vi "SequenceVI.vi"(5 "MSComm":refnum<k7>, 6 "semaphore":T1 caption="信号量", 7 "GUIRefArray":T3[](array[typedef]), 8 "error in":errorcluster, 9 "Slot":T2, 10 "SlotEnable":enum16{"Enable", "Disable"}(ring)=enum."Disable", 11 "QueueArray":variant[](array[variant])) -> (0 "error out":errorcluster)   [LabVIEW 2013]
uses:
  SystemCode/SysControl/Reference.ctl
  SystemCode/SysControl/TestItemsCTL.ctl
  SystemCode/SysControl/Slot.ctl
  SystemCode/SysControl/States.ctl
  SystemCode/DeStateQueue.vi
  SystemCode/EnStateQueue.vi
  SystemCode/ReleaseStateQueue.vi
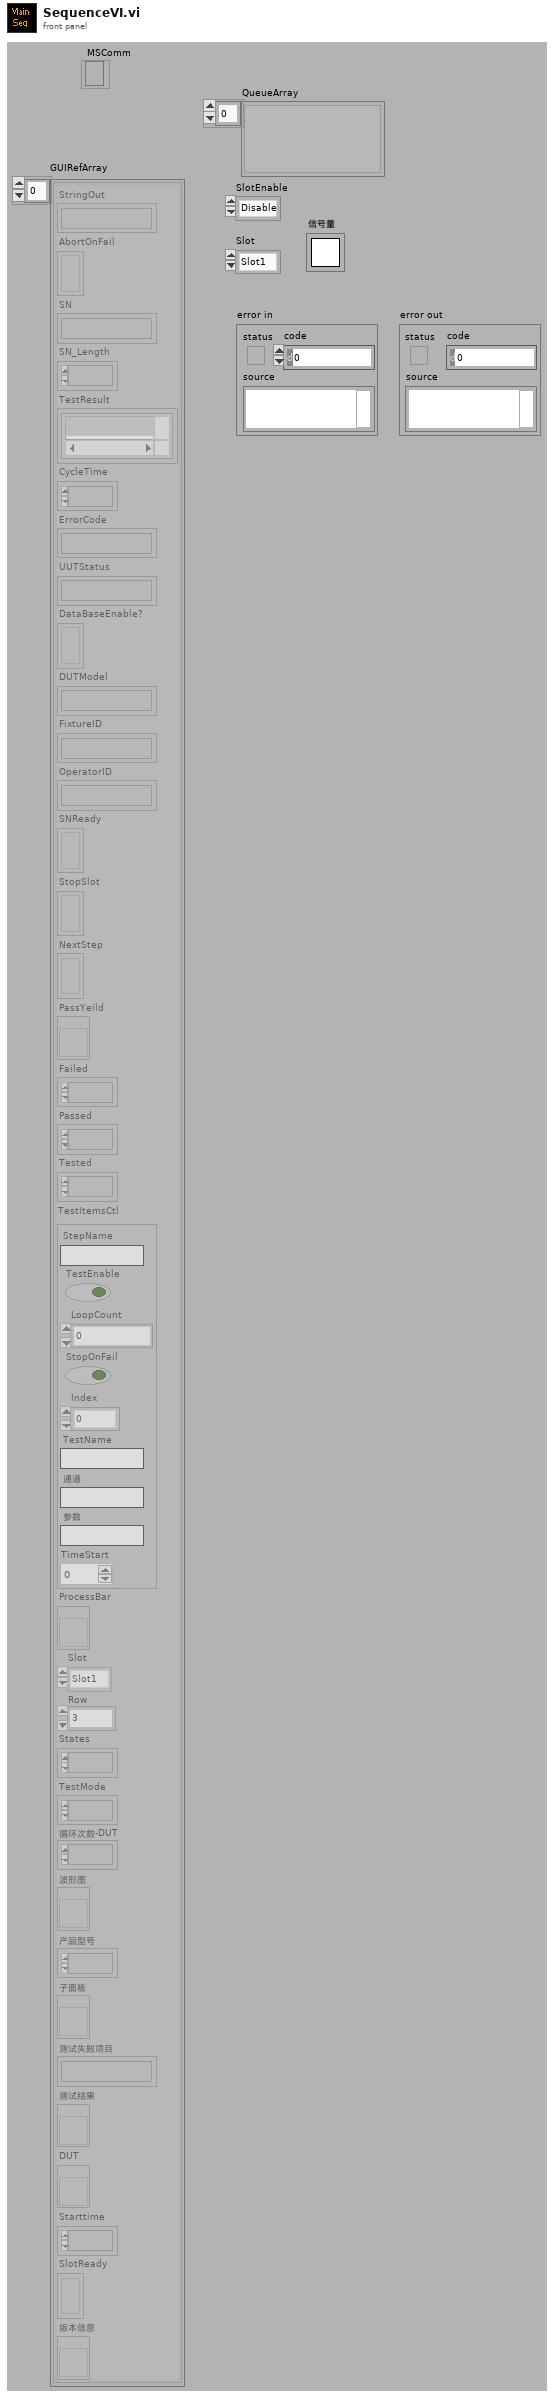
[diagram p1: front panel]
types:
  T1 = typedef "Semaphore RefNum" = refnum<k1>
  T2 = typedef "Slot.ctl" = enum16{"Slot1", "Slot2", "Slot3", "Slot4"}
  T3 = typedef "Reference.ctl" = cluster{"StringOut":refnum<vi>, "AbortOnFail":refnum<vi>, "SN":refnum<vi>, "SN_Length":refnum<vi>, "TestResult":refnum<vi>, "CycleTime":refnum<vi>, "ErrorCode":refnum<vi>, "UUTStatus":refnum<vi>, "DataBaseEnable?":refnum<vi>, "DUTModel":refnum<vi>, "FixtureID":refnum<vi>, "OperatorID":refnum<vi>, "SNReady":refnum<vi>, "StopSlot":refnum<vi>, "NextStep":refnum<vi>, "PassYeild":refnum<vi>, "Failed":refnum<vi>, "Passed":refnum<vi>, "Tested":refnum<vi>, "TestItemsCtl":T4, "ProcessBar":refnum<vi>, "Slot":T2, "Row":u32, "States":refnum<vi>, "TestMode":refnum<vi>, "循环次数-DUT":refnum<vi>, "波形图":refnum<vi>, "产品型号":refnum<vi>, "子面板":refnum<vi>, "测试失败项目":refnum<vi>, "测试结果":refnum<vi>, "DUT":refnum<vi>, "Starttime":refnum<vi>, "SlotReady":refnum<vi>, "版本信息":refnum<vi>}
  T4 = typedef "TestItemsCTL.ctl" = cluster{"StepName":string, "TestEnable":bool, "LoopCount":i32, "StopOnFail":bool, "Index":u32, "TestName":string, "通道":string, "参数":string, "TimeStart":u32}
  T5 = typedef "States.ctl" = enum16{"Init", "PreUUT", "Idle", "SetUp", "TestSequence", "PostUUT", "StopTest", "Debug Mode", "Selection Mode", "Loop Mode", "Error", "Wait"}
  T6 = enum16{"Production Mode", "Selection Mode", "Debug Mode", "Loop Mode"}
  T7 = enum16{"Production Mode", "Selection Mode", "Debug Mode", "Loop Mode", "Stop Test"}
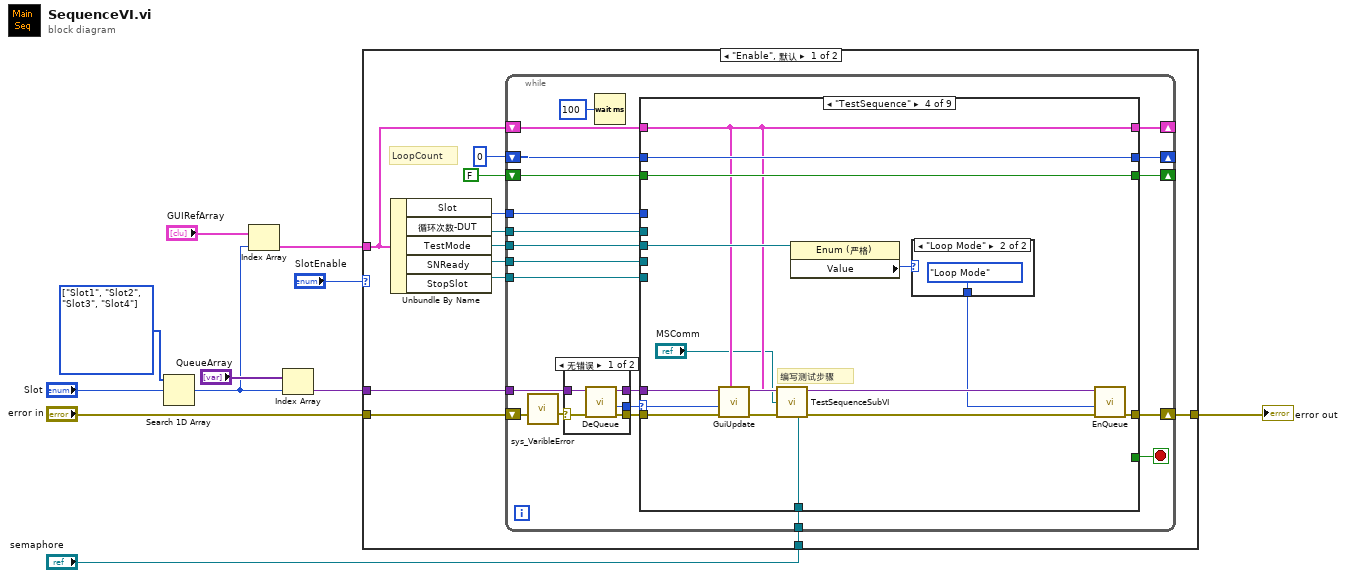
[diagram p0: block diagram]
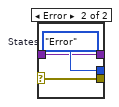
[diagram p2: hidden frame]
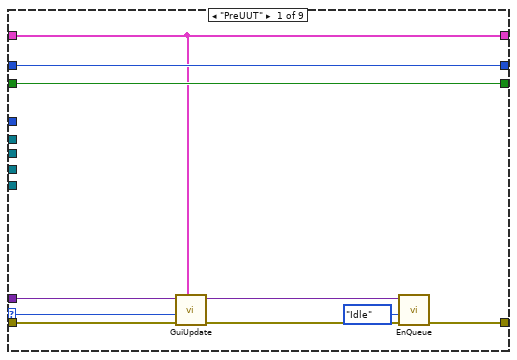
[diagram p3: hidden frame]
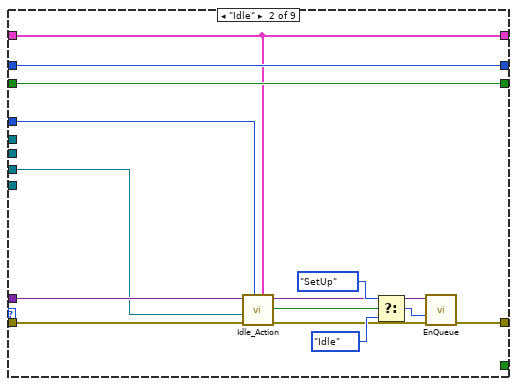
[diagram p4: hidden frame]
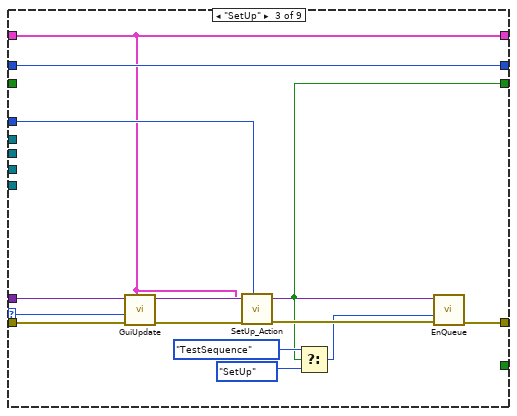
[diagram p5: hidden frame]
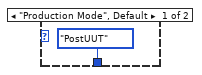
[diagram p6: hidden frame]
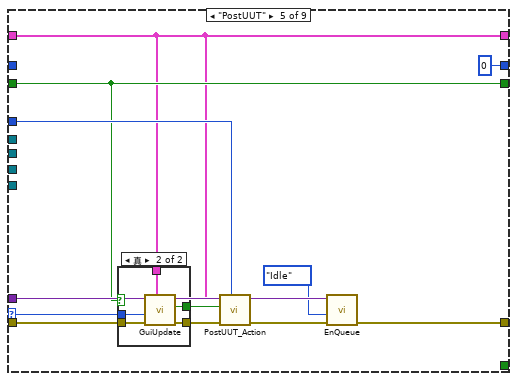
[diagram p7: hidden frame]
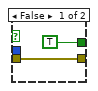
[diagram p8: hidden frame]
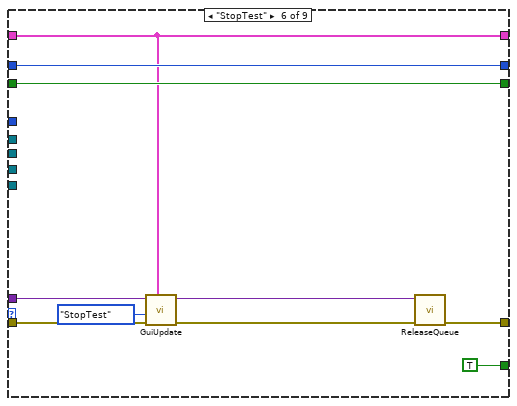
[diagram p9: hidden frame]
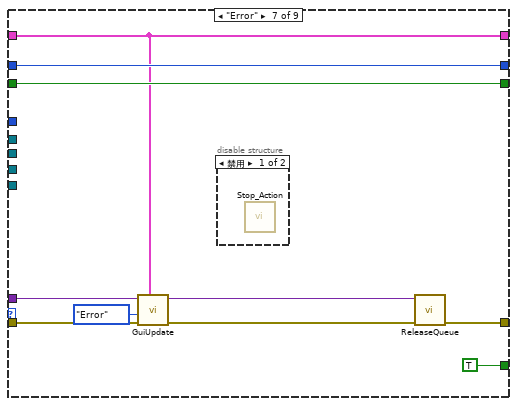
[diagram p10: hidden frame]
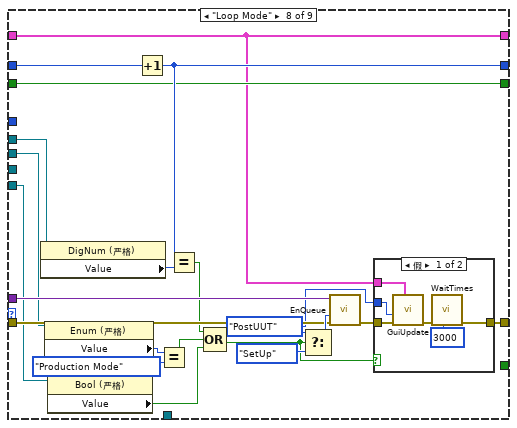
[diagram p12: hidden frame]
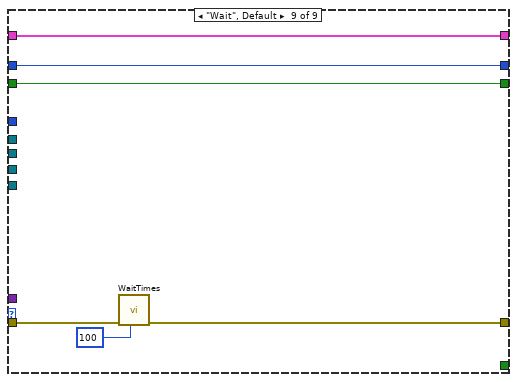
[diagram p14: hidden frame]
diagram:
  w5 = T2[] [enum."Slot1", enum."Slot2", enum."Slot3", enum."Slot4"] items=["Slot1", "Slot2", "Slot3", "Slot4"]
  n1 = Search 1D Array(1D array=w5, element="Slot") -> (index of element=w7:i32)  [unwired: 1 in]
  n2 = Index Array(array="GUIRefArray", index=w7) -> (element=w1:T3)
  n3 = Index Array(array="QueueArray", index=w7) -> (element=w9:variant)
  n4 = case shown="\"Enable\", 默认" "SlotEnable" {
    tunnel: "error in" -> [w19 w175]
    tunnel: [w18 w175] -> w2
    tunnel: w1 -> [w14 _]
    tunnel: w9 -> [w13 _]
    tunnel: "semaphore" -> [w12 _]
    frame "Enable", Default {
      # "LoopCount"
      n5 = Unbundle By Name(w14) -> ("Slot"=w22:T2, "循环次数-DUT"=w20:refnum<vi>, "TestMode"=w21:refnum<vi>, "SNReady"=w16:refnum<vi>, "StopSlot"=w15:refnum<vi>)
      n6 = while {
        shift-right: [w41] -> w18
        shift-left: w19 -> [w26]
        tunnel: w13 -> [w42]
        shift-right: [w37] -> _
        shift-left: w14 -> [w38]
        shift-right: [w35] -> _
        shift-left: 0 -> [w36]
        tunnel: w21 -> [w34]
        tunnel: w22 -> [w33]
        tunnel: w20 -> [w32]
        shift-right: [w31] -> _
        shift-left: FALSE ("ScanSNOK") -> [w30]
        tunnel: w16 -> [w29]
        tunnel: w15 -> [w27]
        tunnel: w12 -> [w24]
        stop <- w43 stop-if-true
        n7 = call "sys_VaribleError.vi"("ErrorIn"=w26) -> ("ErrorOut"=w25:errorcluster)  [unwired: 10 in]
        n8 = case shown="无错误" w25 {
          selector: w25 -> [w49 w50]
          tunnel: [w48 w51] -> w44
          tunnel: [w47 w50] -> w39
          tunnel: [w45 w52] -> w40
          tunnel: w42 -> [w46 w51]
          frame No Error {
            n9 = call-poly "DeQueue.vi"("error in (no error)"=w49, "QueueIn"=w46) -> ("error out"=w47:errorcluster, "State"=w45:T5, "QueueOut"=w48:variant)  [unwired: 7 out]
          }
          frame Error {
            w52 = States."Error"  # States
          }
        }
        n10 = Wait (ms)(milliseconds to wait=u32 100 ("等待时间（毫秒）")) -> ()  [unwired: 1 out]
        n11 = case shown="\"TestSequence\"" w40 {
          selector: w40 -> [w59 _ w84 w96 w111 _ _ _ _]
          tunnel: w44 -> [w56 w73 w87 w100 w115 w131 w140 w161 _]
          tunnel: w39 -> [w61 w67 w85 w97 w112 w127 w136 w154 w174]
          tunnel: [_ _ _ _ _ TRUE TRUE _ _] -> w43
          tunnel: [w57 w71 w86 w99 w113 w128 w137 w155 w172] -> w41
          tunnel: w38 -> [w53 w62 w75 w90 w104 w124 w132 w143 w171]
          tunnel: [w53 w62 w75 w90 w104 w124 w132 w143 w171] -> w37
          tunnel: w36 -> [w60 w69 w83 w93 _ w129 w138 w160 w170]
          tunnel: [w60 w69 w83 w93 0 w129 w138 w158 w170] -> w35
          tunnel: w34 -> [_ _ _ w92 _ _ _ w150 _]
          tunnel: w33 -> [_ w65 w80 _ w108 _ _ _ _]
          tunnel: w32 -> [_ _ _ _ _ _ _ w151 _]
          tunnel: [w54 w64 w76 w91 w106 w125 w134 w149 w169] -> w31
          tunnel: w30 -> [w54 w64 _ w91 w106 w125 w134 w149 w169]
          tunnel: w29 -> [_ w63 _ _ _ _ _ _ _]
          tunnel: w27 -> [_ _ _ _ _ _ _ w148 _]
          tunnel: w24 -> [_ _ _ w89 _ _ _ _ _]
          frame "PreUUT" {
            n12 = call "GuiUpdate.vi"("GuiRef"=w53, "error in"=w61, "States"=w59) -> ("error out"=w58:errorcluster)  [unwired: 2 in, 6 out]
            n13 = call-poly "EnQueue.vi"("error in"=w58, "States"=States."Idle", "QueueIn"=w56) -> ("error out"=w57:errorcluster)  [unwired: 2 in, 6 out]
          }
          frame "Idle" {
            n14 = call "Idle_Action.vi"("GuiRef"=w62, "Slot"=w65, "error in"=w67, "SNReady"=w63) -> ("error out"=w68:errorcluster, "SlotReady"=w66:bool)  [unwired: 6 in]
            n15 = Select(t=States."SetUp" ("EnumOut"), s=w66, f=States."Idle" ("States")) -> (s? t:f=w72:T5)
            n16 = call-poly "EnQueue.vi"("error in"=w68, "States"=w72, "QueueIn"=w73) -> ("error out"=w71:errorcluster)  [unwired: 2 in, 6 out]
          }
          frame "SetUp" {
            n17 = call "GuiUpdate.vi"("GuiRef"=w75, "error in"=w85, "States"=w84) -> ("error out"=w82:errorcluster)  [unwired: 2 in, 6 out]
            n18 = call "SetUp_Action.vi"("Slot"=w80, "error in"=w82, "GuiRef"=w75) -> ("error out"=w81:errorcluster, "ScanSNOK"=w76:bool)  [unwired: 7 in]
            n19 = Select(t=States."TestSequence" ("States"), s=w76, f=States."SetUp" ("States")) -> (s? t:f=w78:T5)
            n20 = call-poly "EnQueue.vi"("error in"=w81, "States"=w78, "QueueIn"=w87) -> ("error out"=w86:errorcluster)  [unwired: 2 in, 6 out]
          }
          frame "TestSequence" {
            # "编写测试步骤"
            n21 = call "GuiUpdate.vi"("GuiRef"=w90, "error in"=w97, "States"=w96) -> ("error out"=w98:errorcluster)  [unwired: 2 in, 6 out]
            n22 = call "TestSequenceSubVI.vi"("GuiRef"=w90, "MSComm"="MSComm", "error in"=w98, "semaphore"=w89) -> ("error out"=w101:errorcluster)  [unwired: 1 in, 10 out]
            n23 = property class="Enum (严格)"(reference=w92) -> ("Value"=w95:T7)  [unwired: 1 in, 2 out]
            n24 = case shown="\"Loop Mode\"" w95 {
              tunnel: [States."PostUUT" ("States") States."Loop Mode" ("States")] -> w94
              frame "Production Mode", Default {
              }
              frame "Loop Mode" {
              }
            }
            n25 = call-poly "EnQueue.vi"("error in"=w101, "States"=w94, "QueueIn"=w100) -> ("error out"=w99:errorcluster)  [unwired: 2 in, 6 out]
          }
          frame "PostUUT" {
            n26 = case shown="真" w106 {
              tunnel: w112 -> [w117 w122]
              tunnel: w111 -> [_ w121]
              tunnel: [w117 w120] -> w110
              tunnel: [TRUE ("PASS/FAIL") w119] -> w107
              tunnel: w104 -> [_ w118]
              frame False {
              }
              frame True {
                n27 = call "GuiUpdate.vi"("GuiRef"=w118, "error in"=w122, "States"=w121) -> ("error out"=w120:errorcluster, "PASS/FAIL"=w119:bool)  [unwired: 2 in, 5 out]
              }
            }
            n28 = call "PostUUT_Action.vi"("Slot"=w108, "error in"=w110, "TestResult"=w107, "GuiRef"=w104) -> ("error out"=w109:errorcluster)  [unwired: 7 in]
            n29 = call-poly "EnQueue.vi"("error in"=w109, "States"=States."Idle", "QueueIn"=w115) -> ("error out"=w113:errorcluster)  [unwired: 2 in, 6 out]
          }
          frame "StopTest" {
            n30 = call "GuiUpdate.vi"("GuiRef"=w124, "error in"=w127, "States"=States."StopTest") -> ("error out"=w123:errorcluster)  [unwired: 2 in, 6 out]
            n31 = call-poly "ReleaseQueue.vi"("error in (no error)"=w123, "QueueIn"=w131) -> ("error out"=w128:errorcluster)  [unwired: 9 out]
          }
          frame "Error" {
            n32 = call "GuiUpdate.vi"("GuiRef"=w132, "error in"=w136, "States"=States."Error") -> ("error out"=w133:errorcluster)  [unwired: 2 in, 6 out]
            n33 = disable-structure shown="禁用" {
              frame Disabled {
                n34 = call "Stop_Action.vi"() -> ()  [unwired: 11 in, 1 out]
              }
              frame Enabled {
              }
            }
            n35 = call-poly "ReleaseQueue.vi"("error in (no error)"=w133, "QueueIn"=w140) -> ("error out"=w137:errorcluster)  [unwired: 9 out]
          }
          frame "Loop Mode" {
            w141 = States."PostUUT" ("States")
            n36 = property class="DigNum (严格)"(reference=w151) -> ("Value"=w159:i32)  [unwired: 1 in, 2 out]
            n37 = property class="Enum (严格)"(reference=w150) -> ("Value"=w153:T7)  [unwired: 1 in, 2 out]
            n38 = property class="Bool (严格)"(reference=w148) -> ("Value"=w145:bool)  [unwired: 1 in, 2 out]
            n39 = Increment(x=w160) -> (x+1=w158:i32)
            n40 = Equal?(x=w153, y=T6."Production Mode") -> (x = y?=w144:bool)
            n41 = Equal?(x=w158, y=w159) -> (x = y?=w146:bool)
            n42 = Compound Arithmetic op=OR(w146, w144, w145) -> (w147:bool)
            n43 = Select(t=w141, s=w147, f=States."SetUp" ("States")) -> (s? t:f=w156:T5)
            n44 = call-poly "EnQueue.vi"("error in"=w154, "States"=w156, "QueueIn"=w161) -> ("error out"=w142:errorcluster)  [unwired: 2 in, 6 out]
            n45 = case shown="假" w147 {
              tunnel: w142 -> [w165 w168]
              tunnel: [w164 w168] -> w155
              tunnel: w143 -> [w162 _]
              tunnel: w141 -> [w163 _]
              frame False {
                n46 = call "GuiUpdate.vi"("GuiRef"=w162, "error in"=w165, "States"=w163) -> ("error out"=w166:errorcluster)  [unwired: 2 in, 6 out]
                n47 = call "WaitTimes.vi"("WaitTimes"=u32 3000, "error in (no error)"=w166) -> ("error out"=w164:errorcluster)  [unwired: 9 in]
              }
              frame True {
              }
            }
          }
          frame "Wait", Default {
            n48 = call "WaitTimes.vi"("WaitTimes"=u32 100, "error in (no error)"=w174) -> ("error out"=w172:errorcluster)  [unwired: 9 out]
          }
        }
      }
    }
    frame "Disable" {
    }
  }
  "error out" <- w2
